vi "Humidity Max Read Single.vi"(8 "error in":errorcluster, 9 "Channel Index":i32=1, 11 "Climate Chamber in":refnum<class "Climate Chamber.lvclass">) -> (0 "error out":errorcluster, 1 "Changed or First Call?":bool, 2 "Humidity Max SP":dbl, 3 "Climate Chamber out":refnum<class "Climate Chamber.lvclass">)   [LabVIEW 2023, in "Climate Chamber.lvclass"]
uses:
  Climate Chamber.lvclass
  Climate Chamber.lvclass/Climate Chamber.ctl
  Low Level Capabilities/Humidity/Humidity Limit/Humidity Limit.lvclass
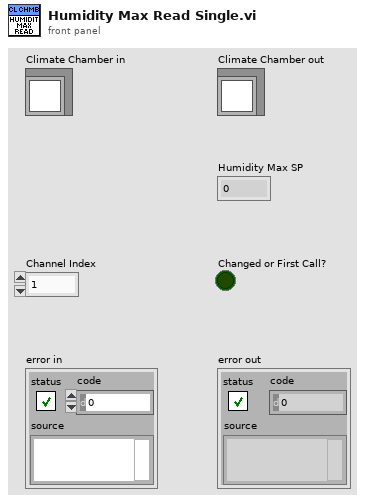
[diagram p1: front panel]
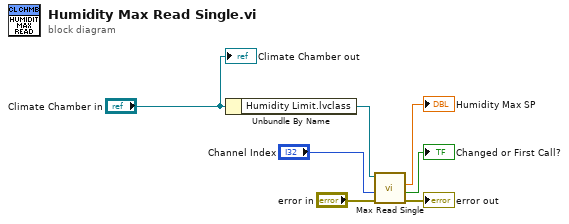
[diagram p0: block diagram]
diagram:
  n1 = Unbundle By Name("Climate Chamber in") -> ("Humidity Limit.lvclass"=w6:refnum<class "Humidity Limit.lvclass">)
  n2 = call-dynamic "Max Read Single.vi"("error in"="error in", "Channel Index"="Channel Index", "Max Humidity Limit in"=w6) -> ("error out"=→"error out":errorcluster, "Changed or First Call?"=→"Changed or First Call?":bool, "Humidity Max SP"=→"Humidity Max SP":dbl)  [unwired: 5 in, 1 out]
  "Climate Chamber out" <- "Climate Chamber in"
